vi "filter_ch.vi"(9 "reset":bool, 10 "filter rate":u16, 11 "filter in":fxp<+/-,16,1> format="%#_16g") -> (3 "filter out":fxp<+/-,16,1> format="%.16g")   [LabVIEW 2021]
doc: "this filter genrate 700 steps at log like shpe.\nfilter rate control the time betwin steps."
uses:
  <instrlib>/_niInstr/Basic Elements/v1/FPGA/Private/Count Up U16.vi
  <instrlib>/_niInstr/Basic Elements/v1/FPGA/niInstr Basic Elements v1 FPGA.lvlib
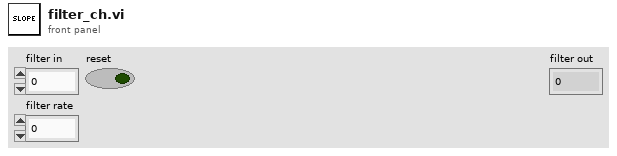
[diagram p1: front panel]
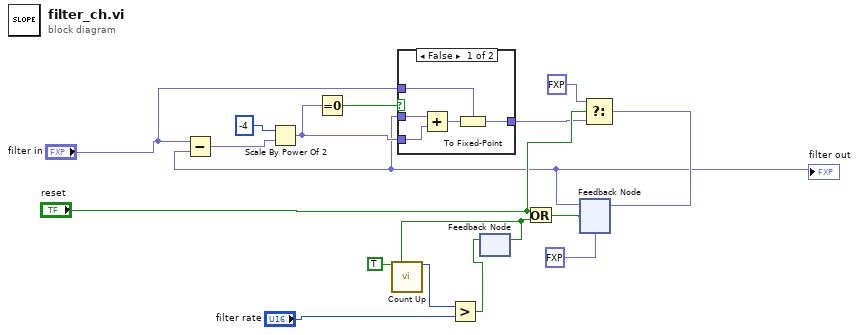
[diagram p0: block diagram]
diagram:
  n1 = feedback #1() -> (w8:bool)  [unwired: 1 in]
  n2 = call-poly <instrlib>:"Count Up.vi"("increment"=TRUE, "reset"=w8) -> ("count out"=w13:u16)  [unwired: 13 in]
  n3 = Greater?(x=w13, y="filter rate") -> (0:w12:bool)
  n4 = feedback-in #1(w12) -> ()
  n5 = Or(x="reset", y=w8) -> (x .or. y?=w7:bool)
  n6 = feedback #2(fxp<+/-,16,1> 0.0 ("Numeric")) -> (w2:fxp<+/-,16,1>)
  "filter out" <- w2
  n7 = Subtract(x="filter in", y=w2) -> (x-y=w16:fxp<+/-,17,2>)
  n8 = Scale By Power Of 2(n=i16 -4, x=w16) -> (x*2^n=w9:fxp<+/-,17,2>)
  n9 = Equal To 0?(x=w9) -> (x = 0?=w14:bool)
  n10 = case shown="False" w14 {
    tunnel: [w20 w23] -> w4
    tunnel: w2 -> [w19 _]
    tunnel: w9 -> [w22 _]
    tunnel: "filter in" -> [w18 w23]
    frame False {
      n11 = Add(x=w19, y=w22) -> (x+y=w21:fxp<+/-,18,3>)
      n12 = To Fixed-Point(fixed-point type=w18, number=w21) -> (fixed-point=w20:fxp<+/-,16,1>)
    }
    frame True {
    }
  }
  n13 = Select(t=fxp<+/-,16,1> 0.0, s="reset", f=w4) -> (s? t:f=w3:fxp<+/-,16,1>)
  n14 = feedback-in #2(w3, w7) -> ()
